vi "ModuleConfigurationMemory.vi"(7 "Operation":T1, 8 "Error In":errorcluster, 10 "task in":refnum<k21>, 11 "Variable In":string) -> (0 "Error Out":errorcluster, 1 "All Variables Out":string[](array[string]), 2 "All Tasks Out":refnum<k21>[](array[refnum]), 3 "Task Out":refnum<k21>, 4 "Found?":bool)   [LabVIEW 2011]
uses:
  Controls/Init-Write-Read.ctl
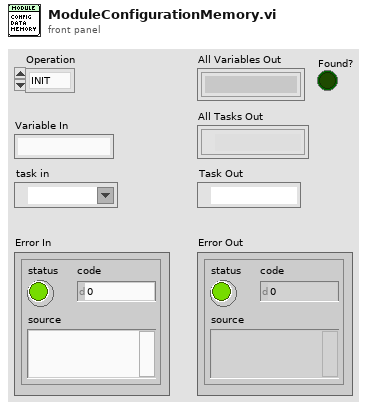
[diagram p1: front panel]
types:
  T1 = typedef "Init-Write-Read.ctl" = enum16{"INIT", "WRITE", "READ", "READ ALL"}
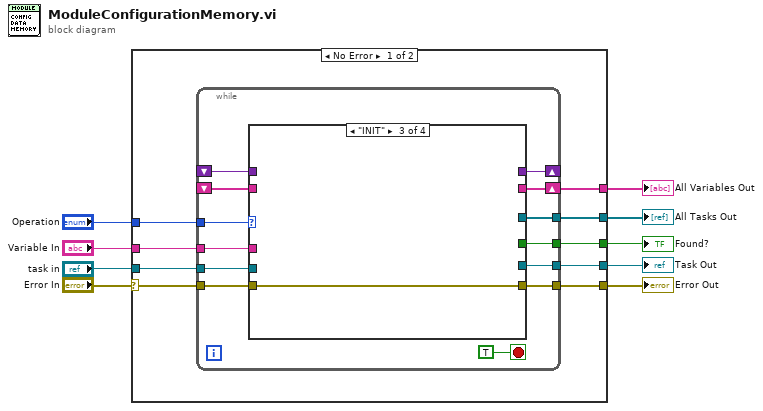
[diagram p0: block diagram]
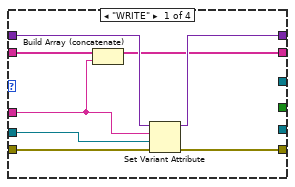
[diagram p2: hidden frame]
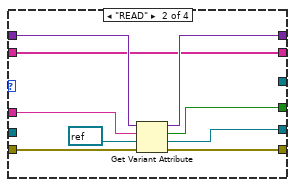
[diagram p3: hidden frame]
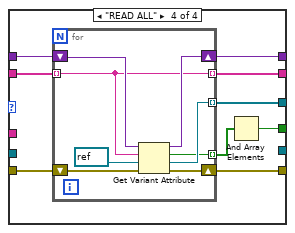
[diagram p4: hidden frame]
diagram:
  n1 = case shown="No Error" "Error In" {
    selector: "Error In" -> [w18 w67]
    tunnel: [w17 w67] -> w2
    tunnel: "Operation" -> [w16 _]
    tunnel: "task in" -> [w15 _]
    tunnel: "Variable In" -> [w14 _]
    tunnel: [w13 _] -> w5
    tunnel: [w12 _] -> w4
    tunnel: [w11 _] -> w3
    tunnel: [w10 _] -> w1
    frame No Error {
      n2 = while {
        tunnel: w18 -> [w31]
        tunnel: [w30] -> w17
        tunnel: w16 -> [w29]
        tunnel: w15 -> [w27]
        shift-right: [w26] -> _
        shift-left: _ -> [w25]
        tunnel: w14 -> [w24]
        shift-right: [w22] -> w13
        shift-left: _ -> [w23]
        tunnel: [w21] -> w12
        tunnel: [w20] -> w11
        tunnel: [w19] -> w10
        stop <- TRUE stop-if-true
        n3 = case shown="\"INIT\"" w29 {
          tunnel: w31 -> [w38 w48 w49 w57]
          tunnel: [w32 w42 w49 w58] -> w30
          tunnel: w27 -> [w39 _ _ _]
          tunnel: [w37 w45 _ w54] -> w26
          tunnel: w25 -> [w36 w46 _ w55]
          tunnel: w24 -> [w34 w47 _ _]
          tunnel: w23 -> [w35 w41 _ w56]
          tunnel: [w33 w41 _ w52] -> w22
          tunnel: [_ w43 _ _] -> w21
          tunnel: [_ _ _ w53] -> w20
          tunnel: [_ w40 _ w50] -> w19
          frame "WRITE" {
            n4 = Build Array (concatenate)(w35, w34) -> (w33:string[])
            n5 = Set Variant Attribute(Variant=w36, name=w34, value=w39, error in=w38) -> (Variant out=w37:variant, error out=w32:errorcluster)  [unwired: 1 out]
          }
          frame "READ" {
            n6 = Get Variant Attribute(Variant=w46, name=w47, default value (empty Variant)=refnum<k21> refnum ("task in"), error in=w48) -> (duplicate Variant=w45:variant, found=w40:bool, value=w43:refnum<k21>, error out=w42:errorcluster)
          }
          frame "INIT" {
          }
          frame "READ ALL" {
            n7 = for {
              tunnel: w56 -> [w60] mode=indexing
              shift-right: [w62] -> w54
              shift-left: w55 -> [w63]
              shift-right: [w65] -> w58
              shift-left: w57 -> [w64]
              tunnel: [w61] -> w53 mode=indexing
              tunnel: [w60] -> w52 mode=indexing
              tunnel: [w59] -> w51 mode=indexing
              n8 = Get Variant Attribute(Variant=w63, name=w60, default value (empty Variant)=refnum<k21> refnum ("task in"), error in=w64) -> (duplicate Variant=w62:variant, found=w59:bool, value=w61:refnum<k21>, error out=w65:errorcluster)
            }
            n9 = And Array Elements(Boolean array=w51) -> (logical AND=w50:bool)
          }
        }
      }
    }
    frame Error {
    }
  }
  "Error Out" <- w2
  "All Variables Out" <- w5
  "Task Out" <- w4
  "All Tasks Out" <- w3
  "Found?" <- w1
